vi "Multi-line.vi"(4 "String":string="a\nb\nc\nd") -> (0 "Array":string[](array[string]))   [LabVIEW 2016]
panel:
  in  "stop":bool
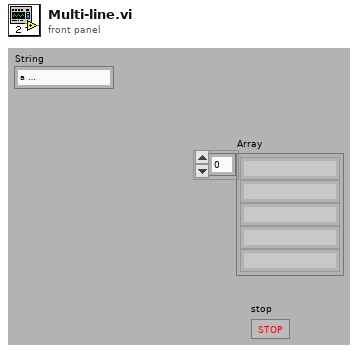
[diagram p1: front panel]
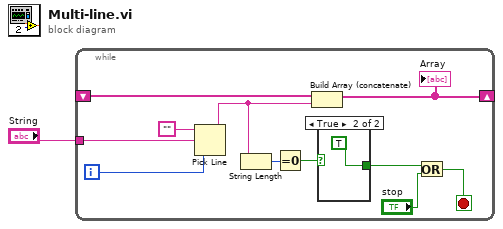
[diagram p0: block diagram]
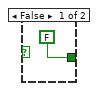
[diagram p2: hidden frame]
diagram:
  n1 = while {
    shift-right: [w10] -> _
    shift-left: _ -> [w11]
    tunnel: "String" -> [w2]
    i -> [w12]
    stop <- w3 stop-if-true
    n2 = Pick Line(string ("")="", multi-line string=w2, line index=w12) -> (output string=w8:string)
    n3 = String Length(string=w8) -> (length=w7:i32)
    n4 = Equal To 0?(x=w7) -> (x = 0?=w6:bool)
    n5 = Build Array (concatenate)(w11, w8) -> (w10:string[])
    "Array" <- w10
    n6 = case shown="True" w6 {
      tunnel: [FALSE TRUE] -> w5
      frame False {
      }
      frame True {
      }
    }
    n7 = Or(x=w5, y="stop") -> (x .or. y?=w3:bool)
  }
